vi "limitted signal.vi"() -> ()   [LabVIEW 2017]
panel:
  out "limitted signal":waveform(dbl)(graph)
  out "main signal":waveform(dbl)[](graph)
  in  "limit":dbl=5.0 format="%0.2f"
  in  "path 3":path
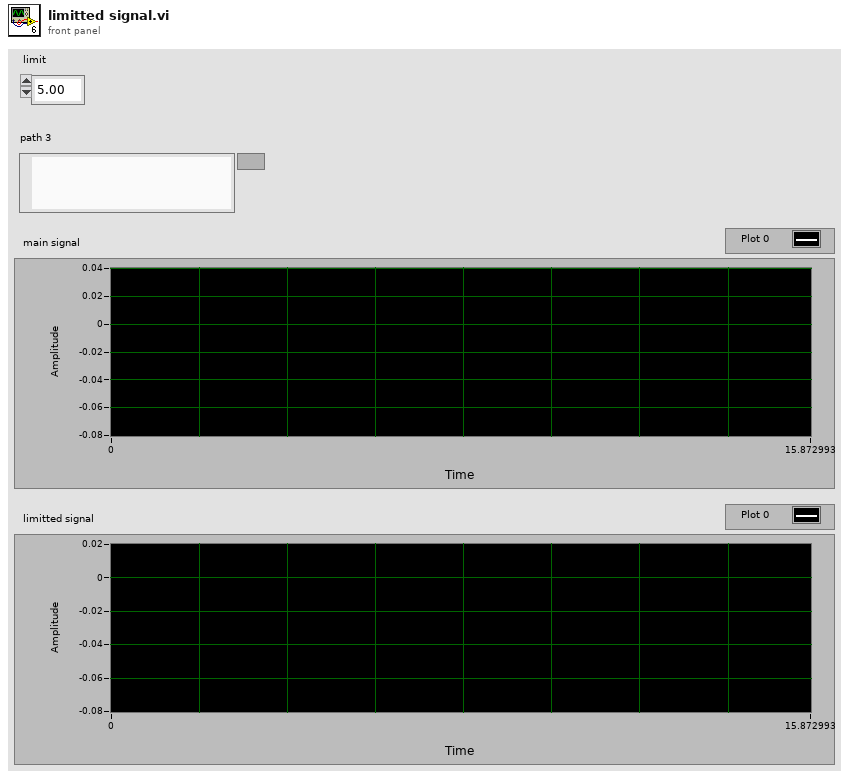
[diagram p1: front panel]
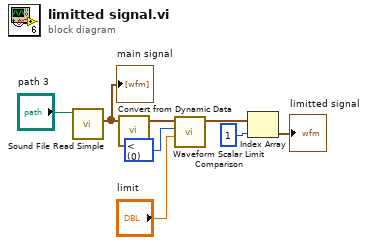
[diagram p0: block diagram]
diagram:
  w6 = u16 0 items=["<", "<=", ">", ">="] ("compare condition")
  n1 = call <vilib>:"Sound File Read Simple.vi"("path"="path 3") -> ("data"=w5:waveform(dbl)[])  [unwired: 7 in, 3 out]
  "main signal" <- w5
  n2 = call "Convert from Dynamic Data"("Dynamic Data Type"=w5) -> ("Waveform"=w4:waveform(dbl))  [unwired: 3 in]
  n3 = call <vilib>:"Waveform Scalar Limit Comparison.vi"("limit"="limit", "compare condition"=w6, "data"=w4) -> ("output waveforms"=w3:waveform(dbl)[])  [unwired: 6 in, 2 out]
  n4 = Index Array(array=w3, index=1) -> (element=→"limitted signal":waveform(dbl))
